vi "Stop Core.vi"(10 "final error code":i32, 11 "[V] User List in":refnum<class "[V] User List.lvclass">) -> (3 "[V] User List out":refnum<class "[V] User List.lvclass">)   [LabVIEW 2020, in "[V] User List.lvlib" / "[V] User List.lvclass"]
doc: "(<B>Filename</B>: Actor Framework.lvlib:Actor.lvclass:Stop Core.vi)\n\nDefines what the actor does before it stops. Use the <B>final error code</B> input to determine whether the actor shut down in response to an error.\n\nBy default, this method passes the Stop message along to all auto-stop nested actors. A descendant class may override this method to define additional behavior, such as shutting down any processes the actor initiated in its override of the Actor Core method."
uses:
  [V] User List.lvclass
  [V] User List.lvclass/[V] User List.ctl
  <vilib>/ActorFramework/Actor/Actor.lvclass
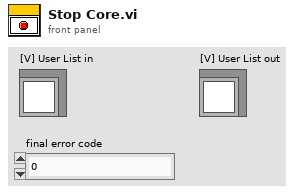
[diagram p1: front panel]
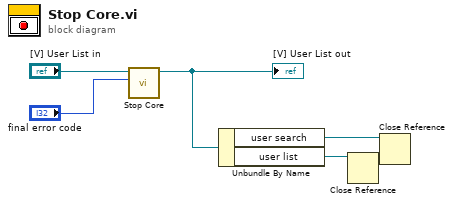
[diagram p0: block diagram]
diagram:
  n1 = call-parent "Stop Core.vi"("final error code"="final error code", "Actor in"="[V] User List in") -> ("Actor out"=w3:refnum<class "[V] User List.lvclass">)  [unwired: 9 in]
  "[V] User List out" <- w3
  n2 = Unbundle By Name(w3) -> ("user search"=w1:refnum<vi>, "user list"=w2:refnum<vi>)
  n3 = Close Reference(reference=w2) -> ()  [unwired: 1 in, 1 out]
  n4 = Close Reference(reference=w1) -> ()  [unwired: 1 in, 1 out]
